vi "lab2_usrp_packet_transceiver.vi"() -> ()   [LabVIEW 2014]
uses:
  <vilib>/addons/Modulation/Analog/support/mod_Set Error Source.vi
  var_stop.vi
  <vilib>/addons/Modulation/Digital/Support/Common/Validators/mod_Generate Filter Coefficients Validate.vi
  <vilib>/addons/Modulation/Digital/General/subVIs/mod_Generate Filter Coefficients.vi
  <vilib>/measure/maspectr.llb/FFT Power Spectrum and PSD for 1 Chan (CDB).vi
  <vilib>/addons/Modulation/Digital/General/MT Apply Matched Filter (Generic).vi
  <vilib>/addons/Modulation/Digital/General/MT Align to Ideal Symbols (Generic).vi
  <instrlib>/niUSRP/niUSRP Fetch Rx Data (CDB Cluster).vi
  <instrlib>/niUSRP/niUSRP Write Tx Data (CDB Cluster).vi
  <vilib>/addons/Modulation/Digital/General/MT Apply Pulse Shaping Filter (Generic).vi
  <vilib>/addons/Modulation/niDMT.lvlib
  <vilib>/measure/NI_MAPro.lvlib
panel:
  in  "Transmit power (db)":dbl
  out "found?":bool
  out "# elements in queue":i32
  out "Spectrum monitor":cluster{"f0":dbl, "df":dbl, "magnitude":dbl[]}(graph)={"f0"=-0.49993781867926873, "df"=0.00012436264146250465, "magnitude"=[]}
  out "RX Constellation Map":cdb[](graph)
  out "valid?":bool
  in  "Gray code?":bool
  in  "Modulation":enum16{"PSK", "QAM"}(ring)=enum."QAM"
  out "Rx String":string
  in  "String":string
  out "packet len":u32
  in  "Send":bool
  in  "filter length (symbols)":i32=8
  in  "filter parameter":dbl=0.5 format="%.2f"
  in  "pulse shaping filter (none)":T1(ring)=enum."Raised Cosine"
  in  "M-PSK (4)":i32=16 caption="M-ARY"
  in  "samples per symbol (16)":i32=4
  out "packet bits length":i32
  in  "number of samples":i64=40000
  out "RX coerced gain":dbl format="%#_6f"
  out "RX coerced carrier frequency":dbl=915000000.0 format="%#_6p"
  out "RX coerced IQ rate":dbl=4000000.0 format="%#_6p"
  in  "RX active antenna":string="RX2"
  in  "RX gain":dbl format="%#_6f"
  in  "RX device names":refnum<k15>="192.168.10.2"
  out "TX coerced gain":dbl format="%#_6f"
  out "TX coerced carrier frequency":dbl=915000000.0 format="%#_6p"
  out "coerced IQ rate":dbl=4000000.0 format="%#_6p"
  in  "TX device names":refnum<k15>="192.168.10.2"
  in  "TX gain":dbl format="%#_6f"
  in  "carrier frequency":dbl=915000000.0 format="%#_6p"
  in  "IQ rate":dbl=800000.0 format="%#_6p"
  in  "stop":bool
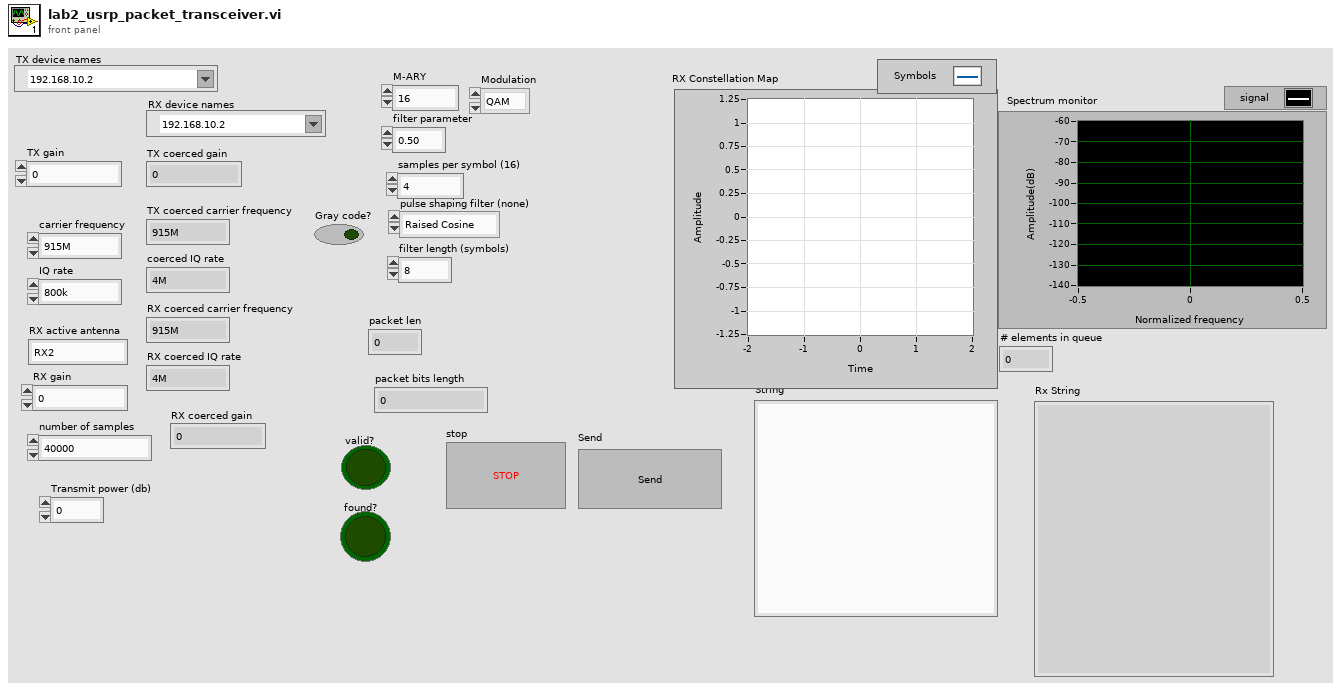
[diagram p1: front panel]
types:
  T1 = enum16{"none", "Raised Cosine", "Root Raised Cos", "Gaussian"}
  T2 = enum16{"FSK", "PSK", "QAM", "MSK", "PAM", "ASK", "CPM"}
  T3 = cluster{"samples per symbol (16)":i32, "symbol map":cdb[], "index map":u32[]}
  T4 = cluster{"samples per symbol (16)":i32, "symbol map":cdb[], i32[]}
  T5 = typedef "niAMT.lvlib/Complex Data Waveform.ctl" = cluster{"t0":dbl, "dt":dbl, "Y":cdb[]}
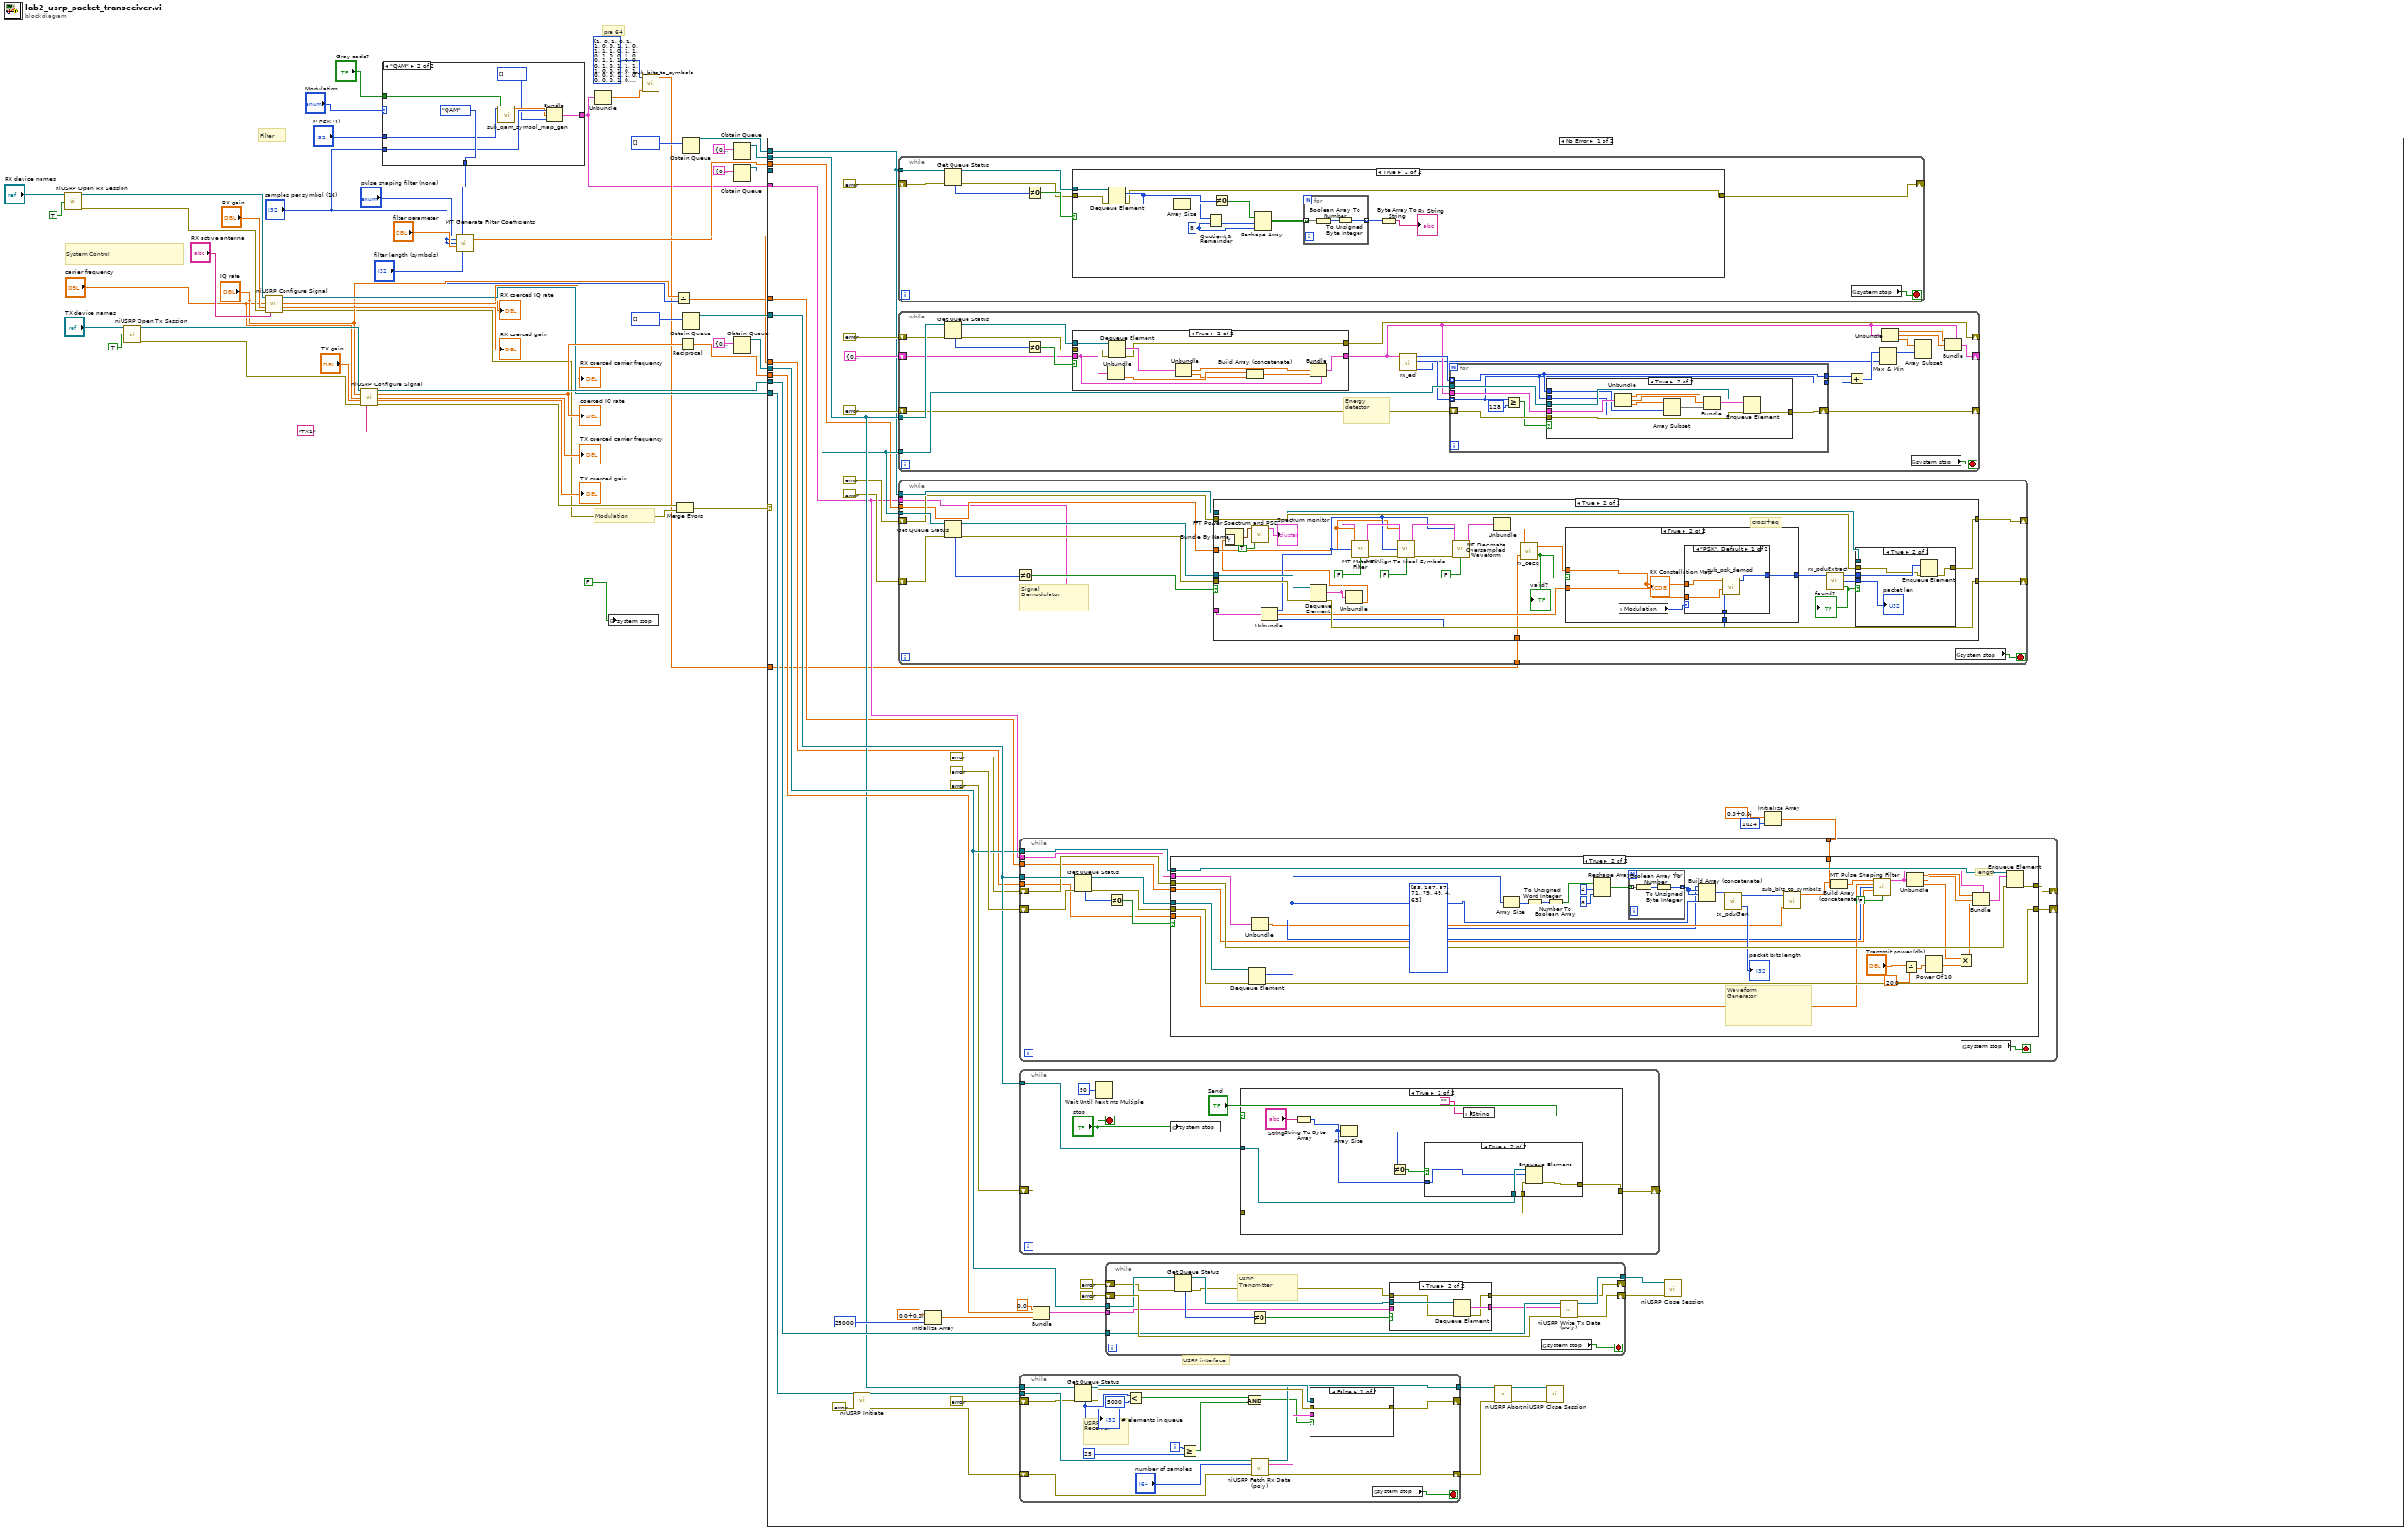
[diagram p0: block diagram]
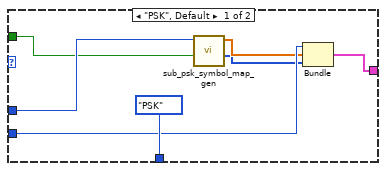
[diagram p2: hidden frame]
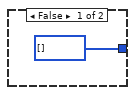
[diagram p5: hidden frame]
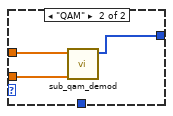
[diagram p6: hidden frame]
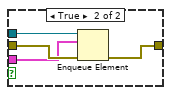
[diagram p10: hidden frame]
diagram:
  # "pre 64"
  # "Modulation"
  # "Filter"
  # "System Control"
  n1 = call <instrlib>:"niUSRP Open Rx Session.vi"("device names"="RX device names", "reset"=TRUE) -> ("session handle out"=w38:refnum<k15>, "error out"=w37:errorcluster)  [unwired: 12 in]
  n2 = call <instrlib>:"niUSRP Open Tx Session.vi"("device names"="TX device names", "reset"=TRUE) -> ("session handle out"=w51:refnum<k15>, "error out"=w50:errorcluster)  [unwired: 12 in]
  n3 = call <instrlib>:"niUSRP Configure Signal.vi"("session handle"=w38, "IQ rate"="IQ rate", "carrier frequency"="carrier frequency", "gain"="RX gain", "error in (no error)"=w37, "active antenna"="RX active antenna") -> ("session handle out"=w29:refnum<k15>, "coerced IQ rate"=→"RX coerced IQ rate":dbl, "coerced carrier frequency"=→"RX coerced carrier frequency":dbl, "coerced gain"=→"RX coerced gain":dbl, "error out"=w13:errorcluster)  [unwired: 5 in]
  n4 = call <instrlib>:"niUSRP Configure Signal.vi"("session handle"=w51, "IQ rate"="IQ rate", "carrier frequency"="carrier frequency", "gain"="TX gain", "error in (no error)"=w50, "active antenna"="TX1") -> ("session handle out"=w42:refnum<k15>, "coerced IQ rate"=w40:dbl, "coerced carrier frequency"=→"TX coerced carrier frequency":dbl, "coerced gain"=→"TX coerced gain":dbl, "error out"=w14:errorcluster)  [unwired: 5 in]
  "coerced IQ rate" <- w40
  n5 = case shown="\"QAM\"" "Modulation" {
    tunnel: [T2."PSK" ("modulation type") T2."QAM" ("modulation type")] -> w8
    tunnel: "M-PSK (4)" -> [w58 w64]
    tunnel: "Gray code?" -> [w57 w65]
    tunnel: "samples per symbol (16)" -> [w56 w63]
    tunnel: [w53 w60] -> w1
    frame "PSK", Default {
      n6 = call "sub_psk_symbol_map_gen.vi"("Gray code?"=w57, "M-PSK"=w58) -> ("index map"=w54:u32[], "symbol map"=w55:cdb[])  [unwired: 8 in]
      n7 = Bundle("samples per symbol (16)"=w56, "symbol map"=w55, "index map"=w54) -> (w53:T3)  [unwired: 1 in]
    }
    frame "QAM" {
      n8 = call "sub_qam_symbol_map_gen.vi"("Gray code?"=w65, "M-QAM"=w64) -> ("symbol map"=w62:cdb[])  [unwired: 9 in]
      n9 = Bundle("samples per symbol (16)"=w63, "symbol map"=w62, i32[] []) -> (w60:T4)  [unwired: 1 in]
    }
  }
  n10 = call <vilib>:"MT Generate Filter Coefficients.vi"("pulse shaping filter (none)"="pulse shaping filter (none)", "modulation type"=w8, "pulse shaping samples per symbol (16)"="samples per symbol (16)", "matched samples per symbol (16)"="samples per symbol (16)", "filter parameter"="filter parameter", "filter length (symbols)"="filter length (symbols)") -> ("pulse shaping filter coefficients"=w19:dbl[], "matched filter coefficients"=w17:dbl[])  [unwired: 7 in, 1 out]
  n11 = Unbundle(w1) -> ("symbol map"=w3:cdb[])  [unwired: 2 out]
  n12 = global write "var_stop.vi" "system stop"(FALSE) -> ()
  n13 = call "sub_bits_to_symbols.vi"("symbol map"=w3, "bits"=i16[] [1, 0, 1, 0, 1, 1, 0, 0, 1, 1, 0, 1, 1, 1, 0, 1, 1, 0, 1, 0, 0, 1, 0, 0, 1, 1, 1, 0, 0, 0, 1, 0, 1, 1, 1, 1, 0, 0, 1, 0, 1, 0, 0, 0, 1, 1, 0, 0, 0, 0, 1, 0, 0, 0, 0, 0, 1, 1, 1, 1, 1, 1, 0, 0] ("preamble(64) 2")) -> ("symbols"=w2:cdb[])  [unwired: 9 in]
  n14 = Divide(x="IQ rate", y="samples per symbol (16)") -> (x/y=w18:dbl)
  n15 = Merge Errors(w14, w13) -> (w12:errorcluster)
  n16 = Reciprocal(x=w40) -> (1/x=w39:dbl)
  n17 = Obtain Queue(element data type=i8[] [] ("output bit stream")) -> (queue out=w24:refnum<queue>)  [unwired: 4 in, 2 out]
  n18 = Obtain Queue(element data type=i16[] []) -> (queue out=w52:refnum<queue>)  [unwired: 4 in, 2 out]
  n19 = Obtain Queue(element data type=cluster{"t0":dbl, "dt":dbl, "Y":cdb[]} {"t0"=0.0, "dt"=0.0, "Y"=[]} ("data")) -> (queue out=w28:refnum<queue>)  [unwired: 4 in, 2 out]
  n20 = Obtain Queue(element data type=cluster{"t0":dbl, "dt":dbl, "Y":cdb[]} {"t0"=0.0, "dt"=0.0, "Y"=[]} ("data")) -> (queue out=w25:refnum<queue>)  [unwired: 4 in, 2 out]
  n21 = Obtain Queue(element data type=cluster{"t0":dbl, "dt":dbl, "Y":cdb[]} {"t0"=0.0, "dt"=1.0, "Y"=[]} ("data")) -> (queue out=w43:refnum<queue>)  [unwired: 4 in, 2 out]
  n22 = case shown="No Error" w12 {
    tunnel: w52 -> [w107 _]
    tunnel: w43 -> [w102 _]
    tunnel: w42 -> [w103 _]
    tunnel: w39 -> [w96 _]
    tunnel: w29 -> [w91 _]
    tunnel: w28 -> [w85 _]
    tunnel: w25 -> [w81 _]
    tunnel: w24 -> [w79 _]
    tunnel: w1 -> [w73 _]
    tunnel: w19 -> [w76 _]
    tunnel: w18 -> [w75 _]
    tunnel: w17 -> [w74 _]
    tunnel: w2 -> [w67 _]
    frame No Error {
      # "USRP interface"
      n23 = call <instrlib>:"niUSRP Initiate.vi"("session handle"=w91, "error in (no error)"=errorcluster {"status"=FALSE, "code"=0, "source"=""}) -> ("session handle out"=w90:refnum<k15>, "error out"=w89:errorcluster)  [unwired: 12 in]
      n24 = while {
        tunnel: w79 -> [w116]
        shift-right: [w109] -> _
        shift-left: errorcluster {"status"=FALSE, "code"=0, "source"=""} ("error out") -> [w115]
        stop <- w114 stop-if-true
        n25 = Get Queue Status(queue=w116, error in (no error)=w115) -> (queue out=w111:refnum<queue>, error out=w110:errorcluster, # elements in queue=w113:i32)  [unwired: 1 in, 5 out]
        n26 = Not Equal To 0?(x=w113) -> (x != 0?=w112:bool)
        n27 = case shown="True" w112 {
          tunnel: w111 -> [_ w128]
          tunnel: w110 -> [w117 w127]
          tunnel: [w117 w120] -> w109
          frame False {
          }
          frame True {
            w123 = 8 ("y")
            n28 = Dequeue Element(queue=w128, error in (no error)=w127) -> (element=w126:i8[], error out=w120:errorcluster)  [unwired: 1 in, 2 out]
            n29 = Array Size(array=w126) -> (size(s)=w125:i32)
            n30 = Quotient & Remainder(x=w125, y=w123) -> (floor(x/y)=w122:i32)  [unwired: 1 out]
            n31 = Not Equal To 0?(x=w126) -> (x != 0?=w124:bool[])
            n32 = Reshape Array(w124, w122, w123) -> (w121:bool[][])
            n33 = for {
              tunnel: w121 -> [w131] mode=indexing
              tunnel: [w130] -> w119 mode=indexing
              n34 = Boolean Array To Number(Boolean array=w131) -> (number=w129:u32)
              n35 = To Unsigned Byte Integer(number=w129) -> (unsigned 8bit integer=w130:u8)
            }
            n36 = Byte Array To String(unsigned byte array=w119) -> (string=→"Rx String":string)
          }
        }
        n37 = global read "var_stop.vi" "system stop"() -> (w114:bool)
      }
      n38 = while {
        tunnel: w85 -> [w223]
        shift-right: [w216] -> _
        shift-left: errorcluster {"status"=FALSE, "code"=0, "source"=""} ("error out") -> [w222]
        shift-right: [w202] -> _
        shift-left: cluster{"t0":dbl, "dt":dbl, "Y":cdb[]} {"t0"=0.0, "dt"=0.0, "Y"=[]} ("data") -> [w217]
        tunnel: w81 -> [w215]
        shift-right: [w214] -> _
        shift-left: errorcluster {"status"=FALSE, "code"=0, "source"=""} ("error out") -> [w213]
        stop <- w212 stop-if-true
        # "Energy\ndetector"
        n39 = Get Queue Status(queue=w223, error in (no error)=w222) -> (queue out=w218:refnum<queue>, error out=w219:errorcluster, # elements in queue=w221:i32)  [unwired: 1 in, 5 out]
        n40 = Not Equal To 0?(x=w221) -> (x != 0?=w220:bool)
        n41 = case shown="True" w220 {
          tunnel: w219 -> [w245 w256]
          tunnel: w218 -> [_ w255]
          tunnel: w217 -> [w244 w250]
          tunnel: [w245 w247] -> w216
          tunnel: [w244 w246] -> w209
          frame False {
          }
          frame True {
            n42 = Unbundle(w250) -> ("Y"=w253:cdb[])  [unwired: 2 out]
            n43 = Dequeue Element(queue=w255, error in (no error)=w256) -> (element=w254:cluster{"t0":dbl, "dt":dbl, "Y":cdb[]}, error out=w247:errorcluster)  [unwired: 1 in, 2 out]
            n44 = Unbundle(w254) -> ("t0"=w249:dbl, "dt"=w248:dbl, "Y"=w252:cdb[])
            n45 = Build Array (concatenate)(w253, w252) -> (w251:cdb[])
            n46 = Bundle(cluster=w250, "t0"=w249, "dt"=w248, "Y"=w251) -> (w246:cluster{"t0":dbl, "dt":dbl, "Y":cdb[]})
          }
        }
        n47 = call "rx_ed.vi"("Wavefrom"=w209) -> ("first pulse"=w199:i32, "length"=w210:i32[], "start index"=w211:i32[])  [unwired: 8 in]
        n48 = for {
          tunnel: w215 -> [w231]
          tunnel: w209 -> [w228]
          shift-right: [w230] -> w214
          shift-left: w213 -> [w229]
          tunnel: w211 -> [w227] mode=indexing
          tunnel: w210 -> [w226] mode=indexing
          tunnel: [w227] -> w205
          tunnel: [w226] -> w204
          n49 = Greater Or Equal?(x=w226, y=128) -> (x >= y?=w224:bool)
          n50 = case shown="True" w224 {
            tunnel: w231 -> [_ w243]
            tunnel: [w232 w242] -> w230
            tunnel: w229 -> [w232 w241]
            tunnel: w228 -> [_ w240]
            tunnel: w227 -> [_ w234]
            tunnel: w226 -> [_ w233]
            frame False {
            }
            frame True {
              n51 = Unbundle(w240) -> ("t0"=w238:dbl, "dt"=w239:dbl, "Y"=w236:cdb[])
              n52 = Array Subset(array=w236, index=w234, length=w233) -> (w235:cdb[])
              n53 = Bundle("t0"=w238, "dt"=w239, w235) -> (w237:cluster{"t0":dbl, "dt":dbl, cdb[]})  [unwired: 1 in]
              n54 = Enqueue Element(queue=w243, element=w237, error in (no error)=w241) -> (error out=w242:errorcluster)  [unwired: 1 in, 2 out]
            }
          }
        }
        n55 = Add(x=w205, y=w204) -> (x+y=w201:i32)
        n56 = Max & Min(x=w201, y=w199) -> (max(x,y)=w200:i32)  [unwired: 1 out]
        n57 = Unbundle(w209) -> ("t0"=w208:dbl, "dt"=w207:dbl, "Y"=w206:cdb[])
        n58 = global read "var_stop.vi" "system stop"() -> (w212:bool)
        n59 = Array Subset(array=w206, index=w200) -> (w203:cdb[])  [unwired: 1 in]
        n60 = Bundle(cluster=w209, "t0"=w208, "dt"=w207, "Y"=w203) -> (w202:cluster{"t0":dbl, "dt":dbl, "Y":cdb[]})
      }
      n61 = while {
        tunnel: w81 -> [w145]
        shift-right: [w139] -> _
        shift-left: errorcluster {"status"=FALSE, "code"=0, "source"=""} ("error out") -> [w144]
        tunnel: w79 -> [w138]
        shift-right: [w137] -> _
        shift-left: errorcluster {"status"=FALSE, "code"=0, "source"=""} ("error out") -> [w136]
        tunnel: w74 -> [w134]
        tunnel: w73 -> [w133]
        tunnel: w67 -> [w132]
        stop <- w135 stop-if-true
        # "Signal \nDemodulator"
        n62 = Get Queue Status(queue=w145, error in (no error)=w144) -> (queue out=w141:refnum<queue>, error out=w140:errorcluster, # elements in queue=w143:i32)  [unwired: 1 in, 5 out]
        n63 = Not Equal To 0?(x=w143) -> (x != 0?=w142:bool)
        n64 = case shown="True" w142 {
          tunnel: w141 -> [_ w178]
          tunnel: w140 -> [w147 w179]
          tunnel: [w147 w177] -> w139
          tunnel: w138 -> [_ w167]
          tunnel: [w146 w166] -> w137
          tunnel: w136 -> [w146 w165]
          tunnel: w134 -> [_ w154]
          tunnel: w133 -> [_ w158]
          tunnel: w132 -> [_ w150]
          frame False {
          }
          frame True {
            # "cross+eq"
            n65 = Unbundle(w158) -> ("samples per symbol (16)"=w157:i32, "symbol map"=w156:cdb[], "index map"=w155:u32[])
            n66 = Dequeue Element(queue=w178, error in (no error)=w179) -> (element=w149:cluster{"t0":dbl, "dt":dbl, "Y":cdb[]}, error out=w177:errorcluster)  [unwired: 1 in, 2 out]
            n67 = Unbundle(w149) -> ("Y"=w148:cdb[])  [unwired: 2 out]
            n68 = Bundle By Name("Y"=w148) -> (w153:waveform(cdb))  [unwired: 1 in]
            n69 = call-poly <vilib>:"FFT Power Spectrum and PSD.vi"("dB On (F)"=TRUE, "time signal"=w153) -> ("Power Spectrum / PSD"=→"Spectrum monitor":cluster{"f0":dbl, "df":dbl, "magnitude":dbl[]})  [unwired: 6 in, 3 out]
            n70 = call-poly <vilib>:"MT Matched Filter.vi"("input complex waveform"=w149, "matched filter coefficients"=w154, "samples per symbol (16)"=w157, "reset? (T)"=FALSE) -> ("output complex waveform"=w176:T5, "error out"=w175:errorcluster)  [unwired: 10 in]
            n71 = call-poly <vilib>:"MT Align To Ideal Symbols.vi"("input complex waveform"=w176, "matched filter coefficients"=w154, "samples per symbol (16)"=w157, "error in (no error)"=w175, "reset? (T)"=FALSE) -> ("output complex waveform"=w173:T5, "error out"=w174:errorcluster)  [unwired: 8 in, 1 out]
            n72 = call <vilib>:"MT Decimate Oversampled Waveform.vi"("input complex waveform"=w173, "decimation factor"=w157, "error in (no error)"=w174, "reset? (T)"=FALSE) -> ("output complex waveform"=w172:T5)  [unwired: 10 in, 1 out]
            n73 = Unbundle(w172) -> ("Y"=w168:cdb[])  [unwired: 2 out]
            n74 = call "rx_ceEq.vi"("preamble"=w150, "symbols"=w168) -> ("valid?"=w163:bool, "eq symbols"=w164:cdb[])
            "valid?" <- w163
            n75 = case shown="True" w163 {
              tunnel: [i8[] [] ("output bit stream") w183] -> w171
              tunnel: w156 -> [_ w184]
              tunnel: w164 -> [_ w181]
              tunnel: w155 -> [_ w182]
              frame False {
              }
              frame True {
                n76 = local read "Modulation"() -> (w185:enum16{"PSK", "QAM"})
                n77 = case shown="\"PSK\", Default" w185 {
                  tunnel: w181 -> [w189 w192]
                  tunnel: w184 -> [w188 w191]
                  tunnel: [w186 w190] -> w183
                  tunnel: w182 -> [w187 _]
                  frame "PSK", Default {
                    n78 = call "sub_psk_demod.vi"("index map"=w187, "symbol map"=w188, "symbol"=w189) -> ("bitstream"=w186:i16[])  [unwired: 8 in]
                  }
                  frame "QAM" {
                    n79 = call "sub_qam_demod.vi"("symbol map"=w191, "symbol"=w192) -> ("bitstream"=w190:i16[])  [unwired: 9 in]
                  }
                }
                "RX Constellation Map" <- w181
              }
            }
            n80 = call "rx_pduExtract.vi"("output bit stream"=w171) -> ("found?"=w170:bool, "packet len"=w162:u32, "ppdu"=w169:i8[])  [unwired: 2 in]
            "found?" <- w170
            n81 = case shown="True" w170 {
              tunnel: w169 -> [_ w196]
              tunnel: w167 -> [_ w198]
              tunnel: [w193 w197] -> w166
              tunnel: w165 -> [w193 w194]
              tunnel: w162 -> [_ w195]
              frame False {
              }
              frame True {
                n82 = Enqueue Element(queue=w198, element=w196, error in (no error)=w194) -> (error out=w197:errorcluster)  [unwired: 1 in, 2 out]
                "packet len" <- w195
              }
            }
          }
        }
        n83 = global read "var_stop.vi" "system stop"() -> (w135:bool)
      }
      n84 = Initialize Array(cdb 0.0+0.0i, 25000 ("dimension size")) -> (w97:cdb[])
      n85 = while {
        tunnel: w107 -> [w361]
        shift-right: [w359] -> _
        shift-left: errorcluster {"status"=FALSE, "code"=0, "source"=""} ("error out") -> [w360]
        stop <- "stop" stop-if-true
        n86 = Wait Until Next ms Multiple(millisecond multiple=u32 50) -> ()  [unwired: 1 out]
        n87 = global write "var_stop.vi" "system stop"("stop") -> ()
        n88 = case shown="True" "Send" {
          tunnel: w361 -> [_ w368]
          tunnel: w360 -> [w364 w367]
          tunnel: [w364 w366] -> w359
          frame False {
          }
          frame True {
            n89 = String To Byte Array(string="String") -> (unsigned byte array=w369:u8[])
            n90 = Array Size(array=w369) -> (size(s)=w365:i32)
            n91 = Not Equal To 0?(x=w365) -> (x != 0?=w370:bool)
            n92 = case shown="True" w370 {
              tunnel: w369 -> [_ w374]
              tunnel: w368 -> [_ w377]
              tunnel: w367 -> [w373 w376]
              tunnel: [w373 w375] -> w366
              frame False {
              }
              frame True {
                n93 = Enqueue Element(queue=w377, element=w374, error in (no error)=w376) -> (error out=w375:errorcluster)  [unwired: 1 in, 2 out]
              }
            }
            n94 = local write "String"("") -> ()
          }
        }
      }
      n95 = while {
        tunnel: w90 -> [w275]
        shift-right: [w263] -> w86
        shift-left: w89 -> [w274]
        tunnel: w85 -> [w272]
        shift-right: [w266] -> _
        shift-left: errorcluster {"status"=FALSE, "code"=0, "source"=""} ("error out") -> [w271]
        tunnel: [w264] -> w87
        i -> [w261]
        stop <- w262 stop-if-true
        # "USRP\nReceiver"
        n96 = Get Queue Status(queue=w272, error in (no error)=w271) -> (queue out=w268:refnum<queue>, error out=w267:errorcluster, # elements in queue=w270:i32)  [unwired: 1 in, 5 out]
        "# elements in queue" <- w270
        n97 = Less?(x=w270, y=5000) -> (x < y?=w259:bool)
        n98 = Greater Or Equal?(x=w261, y=25) -> (x >= y?=w258:bool)
        n99 = And(x=w259, y=w258) -> (x .and. y?=w257:bool)
        n100 = call-poly <instrlib>:"niUSRP Fetch Rx Data (poly).vi"("session handle"=w275, "number of samples"="number of samples", "error in (no error)"=w274) -> ("session handle out"=w264:refnum<k15>, "data"=w265:cluster{"t0":dbl, "dt":dbl, "Y":cdb[]}, "error out"=w263:errorcluster)  [unwired: 9 in, 1 out]
        n101 = case shown="False" w257 {
          tunnel: w268 -> [_ w280]
          tunnel: w267 -> [w276 w279]
          tunnel: [w276 w278] -> w266
          tunnel: w265 -> [_ w277]
          frame False {
          }
          frame True {
            n102 = Enqueue Element(queue=w280, element=w277, error in (no error)=w279) -> (error out=w278:errorcluster)  [unwired: 1 in, 2 out]
          }
        }
        n103 = global read "var_stop.vi" "system stop"() -> (w262:bool)
      }
      n104 = Bundle(0.0, w96, w97) -> (w94:cluster{dbl, dbl, cdb[]})  [unwired: 1 in]
      n105 = while {
        shift-right: [w290] -> w106
        shift-left: errorcluster {"status"=FALSE, "code"=0, "source"=""} ("error out") -> [w288]
        tunnel: [w289] -> w105
        tunnel: w103 -> [w287]
        tunnel: w102 -> [w285]
        shift-right: [w283] -> _
        shift-left: errorcluster {"status"=FALSE, "code"=0, "source"=""} ("error out") -> [w284]
        tunnel: w94 -> [w282]
        stop <- w281 stop-if-true
        # "USRP\nTransmitter"
        n106 = Get Queue Status(queue=w285, error in (no error)=w284) -> (queue out=w292:refnum<queue>, error out=w291:errorcluster, # elements in queue=w294:i32)  [unwired: 1 in, 5 out]
        n107 = Not Equal To 0?(x=w294) -> (x != 0?=w293:bool)
        n108 = case shown="True" w293 {
          tunnel: w292 -> [_ w300]
          tunnel: w291 -> [w295 w299]
          tunnel: [w296 w298] -> w286
          tunnel: [w295 w297] -> w283
          tunnel: w282 -> [w296 _]
          frame False {
          }
          frame True {
            n109 = Dequeue Element(queue=w300, error in (no error)=w299) -> (element=w298:cluster{"t0":dbl, "dt":dbl, "Y":cdb[]}, error out=w297:errorcluster)  [unwired: 1 in, 2 out]
          }
        }
        n110 = global read "var_stop.vi" "system stop"() -> (w281:bool)
        n111 = call-poly <instrlib>:"niUSRP Write Tx Data (poly).vi"("session handle"=w287, "data"=w286, "error in (no error)"=w288) -> ("session handle out"=w289:refnum<k15>, "error out"=w290:errorcluster)  [unwired: 11 in]
      }
      n112 = call <instrlib>:"niUSRP Abort.vi"("session handle"=w87, "error in (no error)"=w86) -> ("session handle out"=w93:refnum<k15>, "error out"=w92:errorcluster)  [unwired: 12 in]
      n113 = call <instrlib>:"niUSRP Close Session.vi"("session handle"=w93, "error in (no error)"=w92) -> ()  [unwired: 13 in, 1 out]
      n114 = call <instrlib>:"niUSRP Close Session.vi"("session handle"=w105, "error in (no error)"=w106) -> ()  [unwired: 13 in, 1 out]
      n115 = Initialize Array(cdb 0.0+0.0i, 1024 ("dimension size")) -> (w68:cdb[])
      n116 = while {
        tunnel: w107 -> [w312]
        shift-right: [w309] -> _
        shift-left: errorcluster {"status"=FALSE, "code"=0, "source"=""} ("error out") -> [w315]
        tunnel: w102 -> [w308]
        shift-right: [w307] -> _
        shift-left: errorcluster {"status"=FALSE, "code"=0, "source"=""} ("error out") -> [w306]
        tunnel: w73 -> [w304]
        tunnel: w76 -> [w303]
        tunnel: w75 -> [w302]
        tunnel: w68 -> [w301]
        stop <- w305 stop-if-true
        n117 = Get Queue Status(queue=w312, error in (no error)=w315) -> (queue out=w310:refnum<queue>, error out=w311:errorcluster, # elements in queue=w314:i32)  [unwired: 1 in, 5 out]
        n118 = Not Equal To 0?(x=w314) -> (x != 0?=w313:bool)
        n119 = case shown="True" w313 {
          tunnel: w311 -> [w317 w354]
          tunnel: w310 -> [_ w353]
          tunnel: [w317 w352] -> w309
          tunnel: w308 -> [_ w347]
          tunnel: [w316 w346] -> w307
          tunnel: w306 -> [w316 w345]
          tunnel: w304 -> [_ w342]
          tunnel: w303 -> [_ w341]
          tunnel: w302 -> [_ w340]
          tunnel: w301 -> [_ w330]
          frame False {
          }
          frame True {
            # "length"
            # "Waveform \nGenerator"
            n120 = Dequeue Element(queue=w353, error in (no error)=w354) -> (element=w326:i16[], error out=w352:errorcluster)  [unwired: 1 in, 2 out]
            n121 = Unbundle(w342) -> ("samples per symbol (16)"=w336:i32, "symbol map"=w328:cdb[])  [unwired: 1 out]
            n122 = Array Size(array=w326) -> (size(s)=w338:i32)
            n123 = To Unsigned Word Integer(number=w338) -> (unsigned 16bit integer=w337:u16)
            n124 = Number To Boolean Array(number=w337) -> (Boolean array=w351:bool[])
            n125 = Reshape Array(w351, 2 ("dimension size"), 8 ("dimension size")) -> (w348:bool[][])
            n126 = for {
              tunnel: w348 -> [w357] mode=indexing
              tunnel: [w355] -> w339 mode=indexing
              n127 = Boolean Array To Number(Boolean array=w357) -> (number=w356:u32)
              n128 = To Unsigned Byte Integer(number=w356) -> (unsigned 8bit integer=w355:u8)
            }
            n129 = Build Array (concatenate)(u8[] [53, 187, 37, 71, 79, 49, 4, 63] ("Array 2"), w339, w339, w326) -> (w344:i16[])
            n130 = call "tx_pduGen.vi"("byte array"=w344) -> ("packet bits length"=→"packet bits length":i32, "pdu"=w329:i32[])  [unwired: 3 in]
            n131 = call "sub_bits_to_symbols.vi"("symbol map"=w328, "bits"=w329) -> ("symbols"=w327:cdb[])  [unwired: 9 in]
            n132 = Build Array (concatenate)(w327, w330) -> (w324:cdb[])
            n133 = call-poly <vilib>:"MT Pulse Shaping Filter.vi"("symbols"=w324, "pulse shaping filter coefficients"=w341, "samples per symbol (16)"=w336, "symbol rate (Hz)"=w340, "reset? (T)"=FALSE) -> ("output complex waveform"=w335:T5)  [unwired: 9 in, 1 out]
            n134 = Divide(x="Transmit power (db)", y=20.0) -> (x/y=w321:dbl)
            n135 = Unbundle(w335) -> ("t0"=w334:dbl, "dt"=w333:dbl, "Y"=w319:cdb[])
            n136 = Power Of 10(x=w321) -> (10^x=w320:dbl)
            n137 = Multiply(x=w319, y=w320) -> (x*y=w318:cdb[])
            n138 = Bundle(cluster=w335, "t0"=w334, "dt"=w333, "Y"=w318) -> (w332:T5)
            n139 = Enqueue Element(queue=w347, element=w332, error in (no error)=w345) -> (error out=w346:errorcluster)  [unwired: 1 in, 2 out]
          }
        }
        n140 = global read "var_stop.vi" "system stop"() -> (w305:bool)
      }
    }
    frame Error {
    }
  }
